vi "Ensure Discovery Service Started.vi"(8 "error in (no error)":errorcluster, 11 "path":path) -> (0 "error out":errorcluster, 3 "key file path":path)   [LabVIEW 2020, in "MeasurementLink Discovery.lvlib"]
uses:
  MeasurementLink Discovery.lvlib
  <vilib>/ErrorRing/Error Ring.xnode
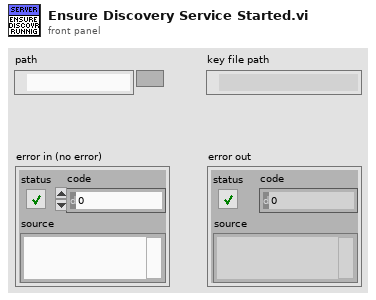
[diagram p1: front panel]
types:
  T1 = enum16{"open", "replace", "create", "open or create", "replace or create", "replace or create with confirmation"}
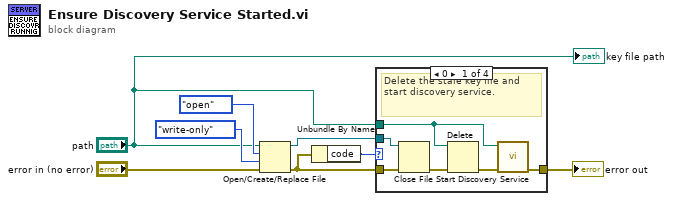
[diagram p0: block diagram]
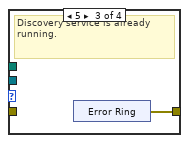
[diagram p3: hidden frame]
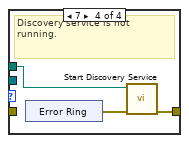
[diagram p4: hidden frame]
diagram:
  n1 = Open/Create/Replace File(file path (use dialog)="path", error in="error in (no error)", operation (0:open)=T1."open", access (0:read/write)=enum16{"read/write", "read-only", "write-only"}."write-only") -> (refnum out=w5:refnum<file>, error out=w3:errorcluster)  [unwired: 2 in, 1 out]
  n2 = Unbundle By Name(w3) -> ("code"=w4:i32)
  n3 = case shown="0" w4 {
    tunnel: w5 -> [w14 _ _ _]
    tunnel: [w11 w15 w16 w20] -> w2
    tunnel: w3 -> [w9 w15 _ _]
    tunnel: "path" -> [w10 _ _ w19]
    frame 0 {
      # "Delete the stale key file and start discovery service."
      n4 = Close File(refnum=w14, error in=w9) -> (error out=w13:errorcluster)  [unwired: 1 out]
      n5 = Delete(path (use dialog)=w10, error in=w13) -> (error out=w12:errorcluster)  [unwired: 3 in, 2 out]
      n6 = call "Start Discovery Service.vi"("error in"=w12, "key file path"=w10) -> ("error out"=w11:errorcluster)  [unwired: 9 in]
    }
    frame 1, Default {
      # "Error occurred in any of the previous node."
    }
    frame 5 {
      # "Discovery service is already running."
      n7 = xnode "Error Ring"() -> ("error out"=w16:errorcluster)
    }
    frame 7 {
      # "Discovery service is not running."
      n8 = xnode "Error Ring"() -> ("error out"=w18:errorcluster)
      n9 = call "Start Discovery Service.vi"("error in"=w18, "key file path"=w19) -> ("error out"=w20:errorcluster)  [unwired: 9 in]
    }
  }
  "error out" <- w2
  "key file path" <- "path"
